vi "test_thcd401.vi"(10 "port":u16=101, 11 "address":string="192.168.24.205") -> (0 "error out":errorcluster)   [LabVIEW 2019]
panel:
  out "mode_array":i32[](array[numeric])
  out "value_array":dbl[](array[numeric])
  in  "wait":u32=1000 caption="ms"
  out "status_init":bool
  out "N":i32
  out "status_read":bool
  in  "stop":bool
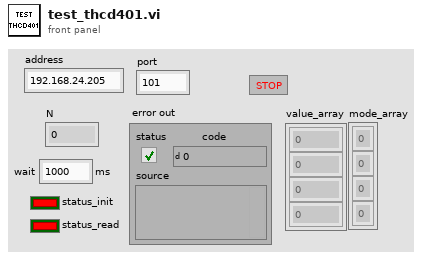
[diagram p1: front panel]
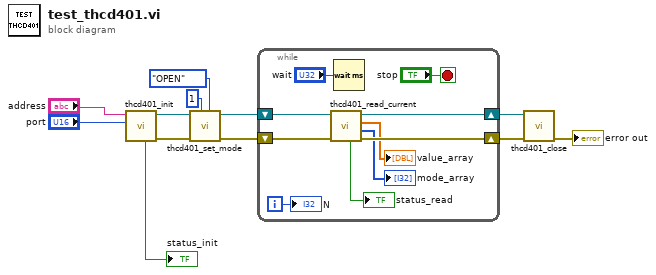
[diagram p0: block diagram]
diagram:
  n1 = call "thcd401_init.vi"("port"="port", "address"="address") -> ("error out"=w3:errorcluster, "conn_id"=w6:refnum<k5>, "status"=→"status_init":bool)  [unwired: 7 in]
  n2 = call "thcd401_set_mode.vi"("mode"=enum16{"AUTO", "OPEN", "CLOSE"}."OPEN", "channel"=u8 1, "error in"=w3, "conn_id_in"=w6) -> ("error out"=w4:errorcluster, "conn_id_out"=w5:refnum<k5>)  [unwired: 5 in, 1 out]
  n3 = while {
    shift-right: [w18] -> w10
    shift-left: w5 -> [w21]
    shift-right: [w17] -> w12
    shift-left: w4 -> [w20]
    i -> [w19]
    stop <- "stop" stop-if-true
    n4 = call "thcd401_read_current.vi"("error in"=w20, "conn_id_in"=w21) -> ("error out"=w17:errorcluster, "mode_array"=→"mode_array":i32[], "value_array"=→"value_array":dbl[], "conn_id_out"=w18:refnum<k5>, "status"=→"status_read":bool)  [unwired: 5 in]
    n5 = Wait (ms)(milliseconds to wait="wait") -> ()  [unwired: 1 out]
    "N" <- w19
  }
  n6 = call "thcd401_close.vi"("error in"=w12, "conn_id"=w10) -> ("error out"=→"error out":errorcluster)  [unwired: 8 in, 1 out]
